vi "File and Folder Info.vi"(8 "error in (no error)":errorcluster, 11 "Path Cluster":T1) -> (0 "error out":errorcluster, 3 "Path Cluster 2":T1)   [LabVIEW 2022 SP3]
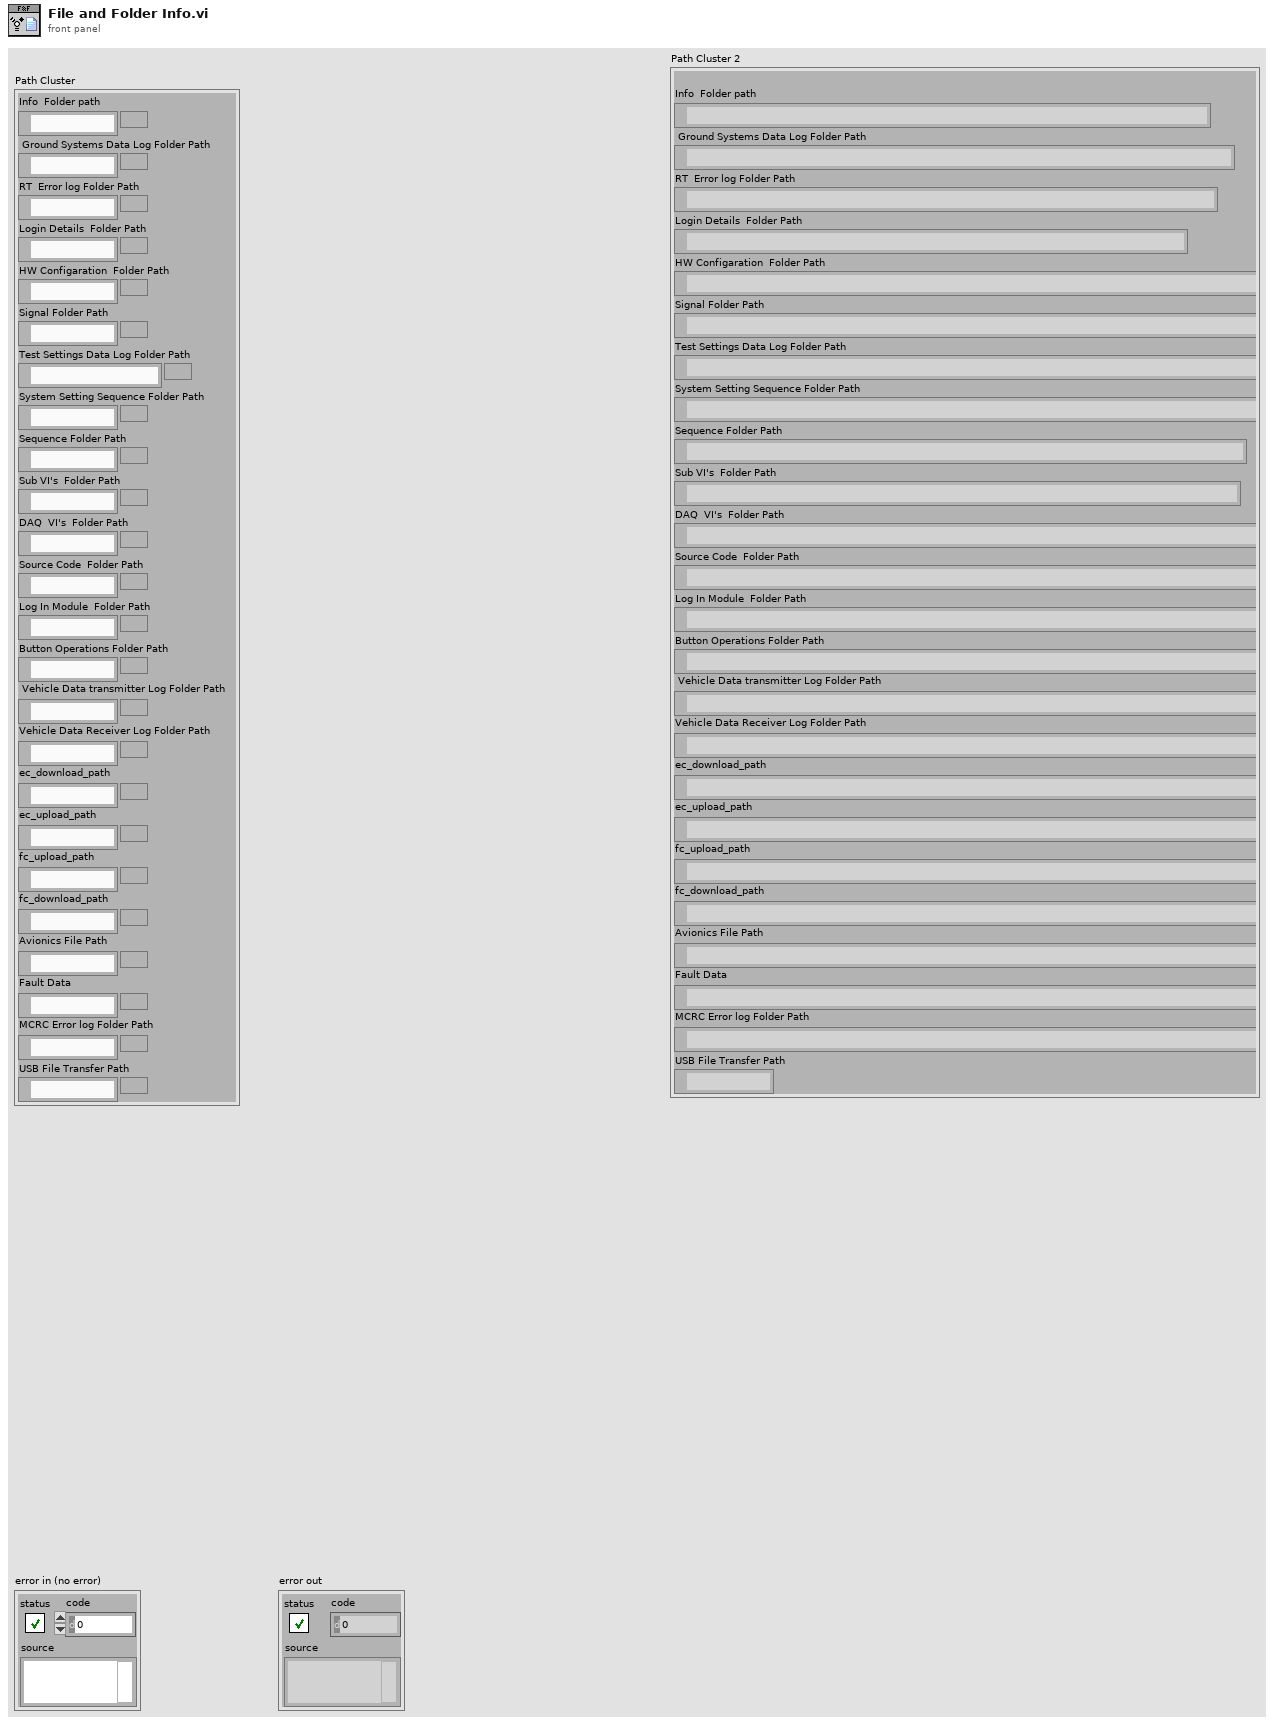
[diagram p1: front panel]
types:
  T1 = cluster{"Info  Folder path":path, " Ground Systems Data Log Folder Path ":path, "RT  Error log Folder Path":path, "Login Details  Folder Path":path, "HW Configaration  Folder Path":path, "Signal Folder Path":path, "Test Settings Data Log Folder Path ":path, "System Setting Sequence Folder Path":path, "Sequence Folder Path":path, "Sub VI's  Folder Path":path, "DAQ  VI's  Folder Path":path, "Source Code  Folder Path":path, "Log In Module  Folder Path ":path, "Button Operations Folder Path":path, "Vehicle Data transmitter Log Folder Path ":path, "Vehicle Data Receiver Log Folder Path ":path, "ec_download_path":path, "ec_upload_path":path, "fc_upload_path":path, "fc_download_path":path, "Avionics File Path ":path, "Fault Data":path, "MCRC Error log Folder Path":path, "USB File Transfer Path":path}
  T2 = enum32{"invalid app kind", "Development System", "Run Time System", "Student Edition", "Embedded LabVIEW", "Evaluation", "Custom"}
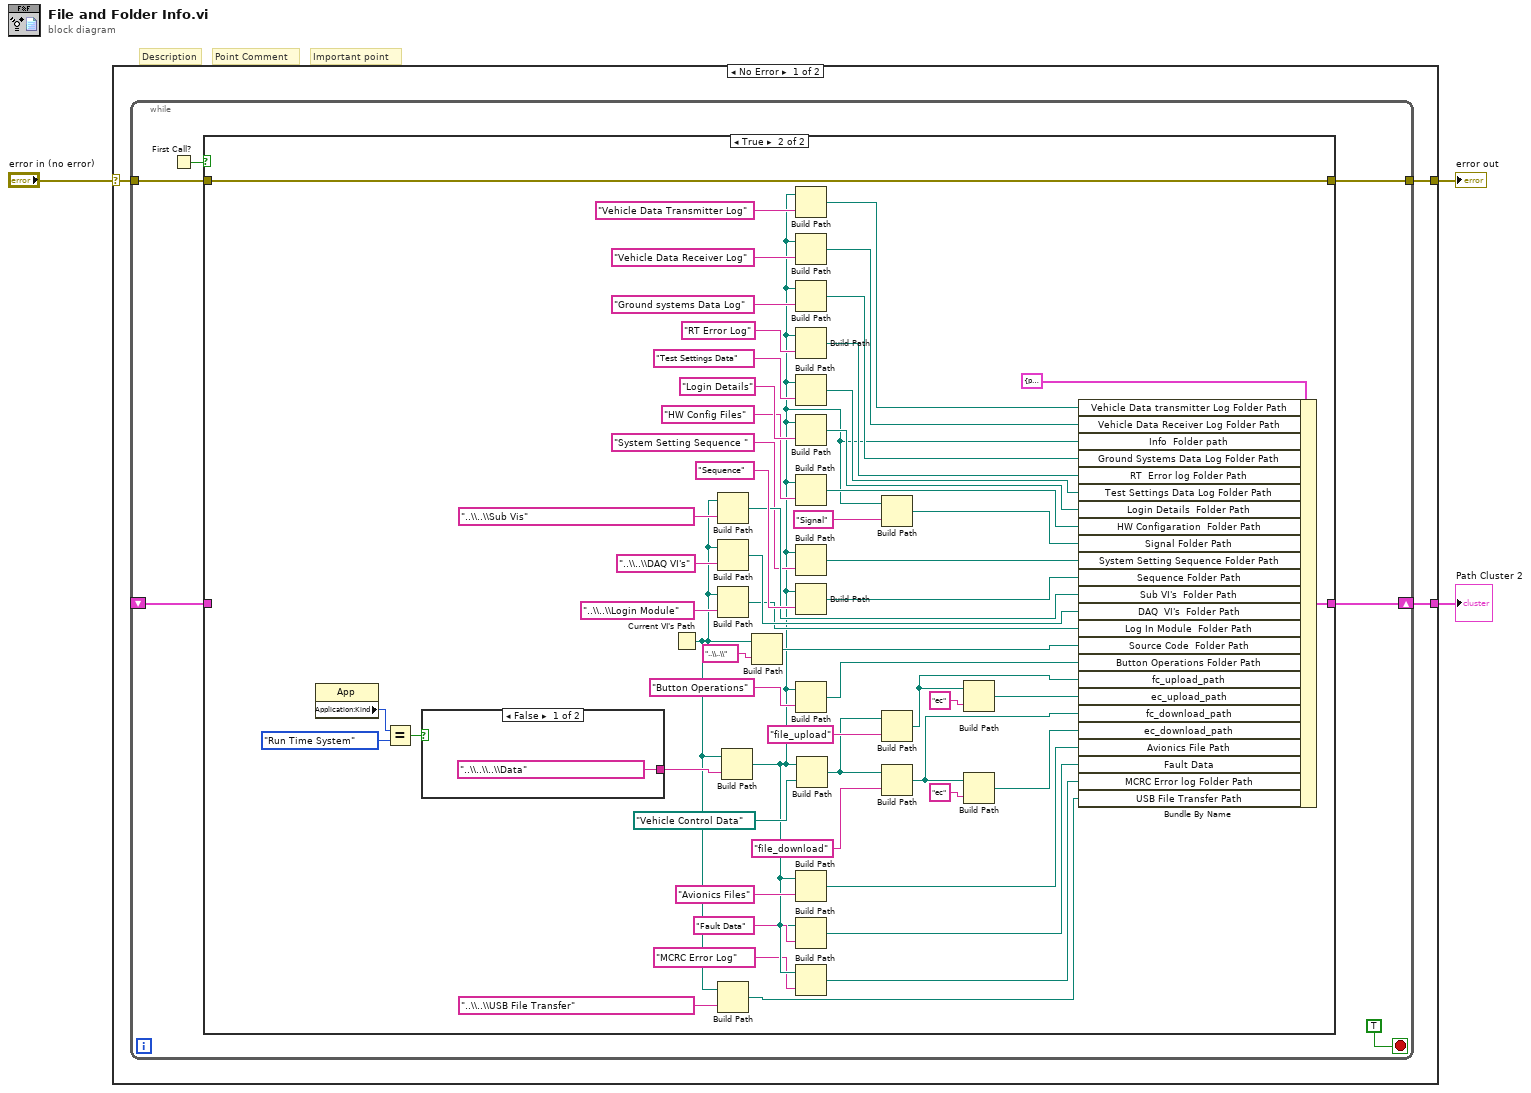
[diagram p0: block diagram]
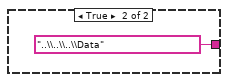
[diagram p3: hidden frame]
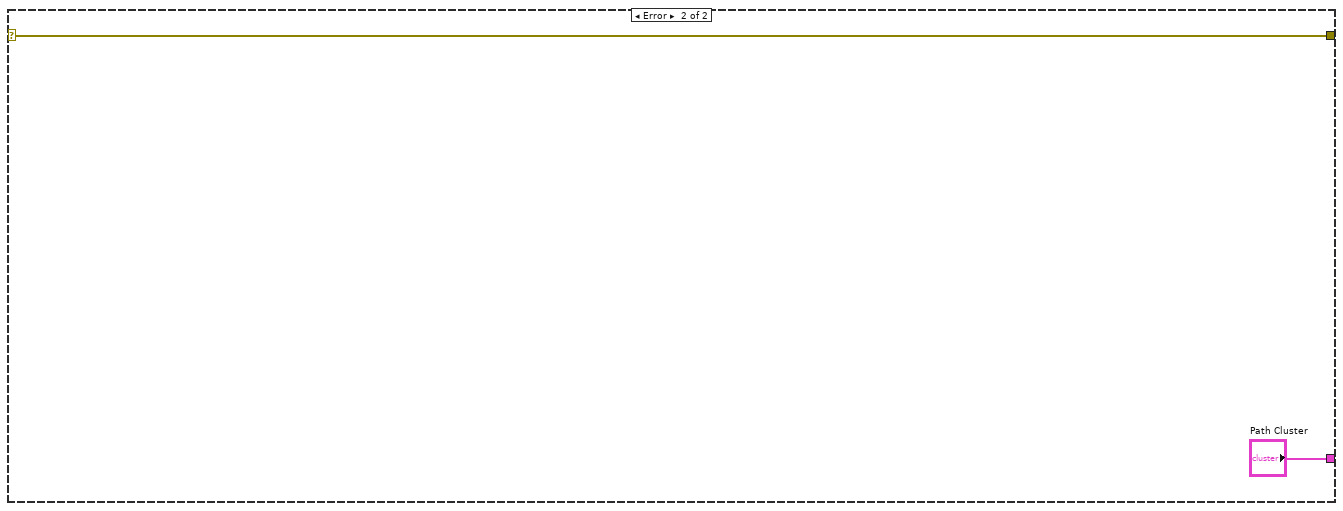
[diagram p4: hidden frame]
diagram:
  # "Point Comment"
  # "Important point"
  # "Description"
  n1 = case shown="No Error" "error in (no error)" {
    selector: "error in (no error)" -> [w6 w75]
    tunnel: [w5 w75] -> w2
    tunnel: [w4 "Path Cluster"] -> w1
    frame No Error {
      n2 = while {
        tunnel: w6 -> [w9]
        tunnel: [w11] -> w5
        shift-right: [w8] -> w4
        shift-left: _ -> [w7]
        stop <- TRUE stop-if-true
        n3 = First Call?() -> (First Call?: T/F=w12:bool)
        n4 = case shown="True" w12 {
          tunnel: w9 -> [w14 w65]
          tunnel: [w14 w65] -> w11
          tunnel: [w13 w66] -> w8
          tunnel: w7 -> [w13 _]
          frame False {
            # "Get Paths"
          }
          frame True {
            n5 = property class="App"() -> ("Application:Kind"=w70:T2)  [unwired: 2 in, 2 out]
            n6 = Equal?(x=w70, y=T2."Run Time System") -> (x = y?=w47:bool)
            n7 = case shown="False" w47 {
              tunnel: ["..\\..\\..\\Data" ("name or relative path") "..\\..\\..\\Data" ("name or relative path")] -> w71
              frame False {
              }
              frame True {
              }
            }
            n8 = Current VI's Path() -> (path=w16:path)
            n9 = Build Path(base path=w16, name or relative path="..\\..\\Sub Vis") -> (appended path=w51:path)
            n10 = Build Path(base path=w16, name or relative path="..\\..\\DAQ VI's") -> (appended path=w45:path)
            n11 = Build Path(base path=w16, name or relative path="..\\..\\Login Module") -> (appended path=w43:path)
            n12 = Build Path(base path=w16, name or relative path="..\\..\\USB File Transfer") -> (appended path=w15:path)
            n13 = Build Path(base path=w16, name or relative path=w71) -> (appended path=w29:path)
            n14 = Build Path(base path=w16, name or relative path="..\\..\\") -> (appended path=w41:path)
            n15 = Build Path(base path=w29, name or relative path="Vehicle Data Transmitter Log") -> (appended path=w34:path)
            n16 = Build Path(base path=w29, name or relative path="Vehicle Data Receiver Log") -> (appended path=w35:path)
            n17 = Build Path(base path=w29, name or relative path="Ground systems Data Log") -> (appended path=w59:path)
            n18 = Build Path(base path=w29, name or relative path="RT Error Log") -> (appended path=w68:path)
            n19 = Build Path(base path=w29, name or relative path="Test Settings Data") -> (appended path=w57:path)
            n20 = Build Path(base path=w29, name or relative path="Login Details") -> (appended path=w55:path)
            n21 = Build Path(base path=w29, name or relative path="HW Config Files") -> (appended path=w53:path)
            n22 = Build Path(base path=w29, name or relative path="System Setting Sequence ") -> (appended path=w48:path)
            n23 = Build Path(base path=w29, name or relative path="Sequence") -> (appended path=w50:path)
            n24 = Build Path(base path=w29, name or relative path="Button Operations") -> (appended path=w39:path)
            n25 = Build Path(base path=w29, name or relative path="Avionics Files") -> (appended path=w32:path)
            n26 = Build Path(base path=w29, name or relative path="Fault Data") -> (appended path=w30:path)
            n27 = Build Path(base path=w29, name or relative path="MCRC Error Log") -> (appended path=w27:path)
            n28 = Build Path(base path=w29, name or relative path=path "Vehicle Control Data") -> (appended path=w25:path)
            n29 = Build Path(base path=w29, name or relative path="Signal") -> (appended path=w52:path)
            n30 = Build Path(base path=w25, name or relative path="file_upload") -> (appended path=w21:path)
            n31 = Build Path(base path=w25, name or relative path="file_download") -> (appended path=w19:path)
            n32 = Build Path(base path=w21, name or relative path="ec") -> (appended path=w20:path)
            n33 = Build Path(base path=w19, name or relative path="ec") -> (appended path=w18:path)
            n34 = Bundle By Name(cluster=T1 {"Info  Folder path"=path "", " Ground Systems Data Log Folder Path "=path "", "RT  Error log Folder Path"=path "", "Login Details  Folder Path"=path "", "HW Configaration  Folder Path"=path "", "Signal Folder Path"=path "", "Test Settings Data Log Folder Path "=path "", "System Setting Sequence Folder Path"=path "", "Sequence Folder Path"=path "", "Sub VI's  Folder Path"=path "", "DAQ  VI's  Folder Path"=path "", "Source Code  Folder Path"=path "", "Log In Module  Folder Path "=path "", "Button Operations Folder Path"=path "", "Vehicle Data transmitter Log Folder Path "=path "", "Vehicle Data Receiver Log Folder Path "=path "", "ec_download_path"=path "", "ec_upload_path"=path "", "fc_upload_path"=path "", "fc_download_path"=path "", "Avionics File Path "=path "", "Fault Data"=path "", "MCRC Error log Folder Path"=path "", "USB File Transfer Path"=path ""} ("Path Cluster"), "Vehicle Data transmitter Log Folder Path"=w34, "Vehicle Data Receiver Log Folder Path"=w35, "Info  Folder path"=w29, "Ground Systems Data Log Folder Path"=w59, "RT  Error log Folder Path"=w68, "Test Settings Data Log Folder Path"=w57, "Login Details  Folder Path"=w55, "HW Configaration  Folder Path"=w53, "Signal Folder Path"=w52, "System Setting Sequence Folder Path"=w48, "Sequence Folder Path"=w50, "Sub VI's  Folder Path"=w51, "DAQ  VI's  Folder Path"=w45, "Log In Module  Folder Path"=w43, "Source Code  Folder Path"=w41, "Button Operations Folder Path"=w39, "fc_upload_path"=w21, "ec_upload_path"=w20, "fc_download_path"=w19, "ec_download_path"=w18, "Avionics File Path"=w32, "Fault Data"=w30, "MCRC Error log Folder Path"=w27, "USB File Transfer Path"=w15) -> (w66:T1)
          }
        }
      }
    }
    frame Error {
    }
  }
  "error out" <- w2
  "Path Cluster 2" <- w1
